vi "String to I64.vi"(8 "error in (no error)":errorcluster, 11 "String to Convert":string) -> (0 "error out":errorcluster, 3 "I64 Value":i64 format="%.0g")   [LabVIEW 2023, in "HAF.lvlib"]
doc: "Convert a String representation of a 64-bit Integer to an actual 64-bit Integer."
uses:
  HAF.lvlib
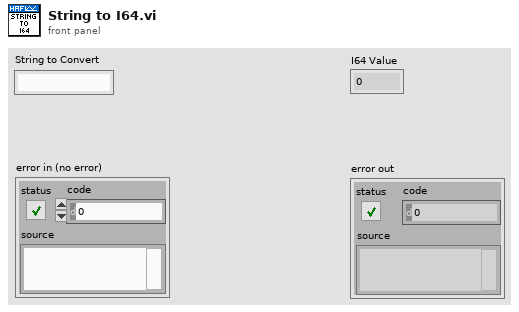
[diagram p1: front panel]
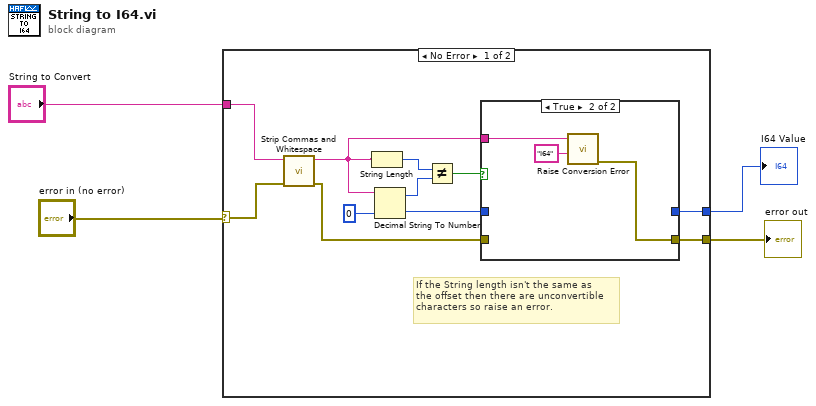
[diagram p0: block diagram]
diagram:
  n1 = case shown="No Error" "error in (no error)" {
    selector: "error in (no error)" -> [w14 w21]
    tunnel: "String to Convert" -> [w15 _]
    tunnel: [w6 w21] -> w2
    tunnel: [w5 _] -> w1
    frame No Error {
      # "If the String length isn't the same as\nthe offset then there are unconvertible\ncharacters so raise an error."
      n2 = call "Strip Commas and Whitespace.vi"("error in (no error)"=w14, "String to Strip"=w15) -> ("error out"=w7:errorcluster, "Clean String"=w9:string)  [unwired: 8 in]
      n3 = String Length(string=w9) -> (length=w11:i32)
      n4 = Decimal String To Number(string=w9, default (0L)=i64 0 ("default (0 I32)")) -> (offset past number=w12:i32, number=w8:i64)  [unwired: 1 in]
      n5 = Not Equal?(x=w11, y=w12) -> (x != y?=w10:bool)
      n6 = case shown="True" w10 {
        tunnel: w9 -> [_ w20]
        tunnel: w8 -> [w17 _]
        tunnel: w7 -> [w16 _]
        tunnel: [w16 w18] -> w6
        tunnel: [w17 _] -> w5
        frame False {
        }
        frame True {
          n7 = call "Raise Conversion Error.vi"("Data Type Attempted"="I64", "String in Error"=w20) -> ("error out"=w18:errorcluster)  [unwired: 9 in]
        }
      }
    }
    frame Error {
    }
  }
  "I64 Value" <- w1
  "error out" <- w2
